vi "Apply Module Limits Fixed.vi"(8 "error in":errorcluster, 11 "3300 in":refnum<class "3300.lvclass">) -> (0 "error out":errorcluster, 3 "3300 out":refnum<class "3300.lvclass">)   [LabVIEW 2019, in "3300.lvlib" / "3300.lvclass"]
uses:
  Library/3300.lvclass
  C:/Users/Public/Documents/Development/builds/Instruments/Electronic Load.lvlibp/Library/Electronic Load.lvclass
  builds/Instruments/Electronic Load.lvlibp/Private/GUI/Read Settings_Ref.vi
  Module Support/Access Module Limits.vi
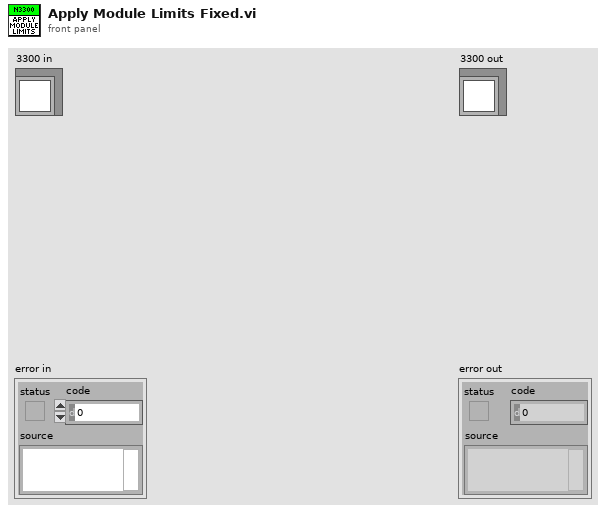
[diagram p1: front panel]
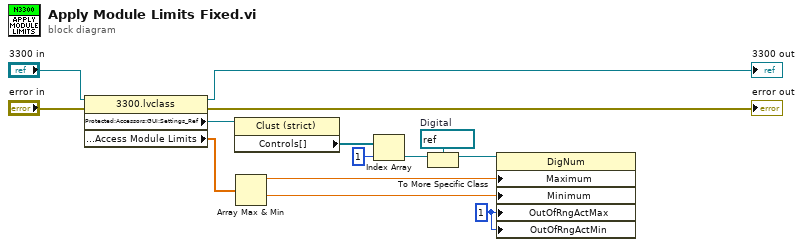
[diagram p0: block diagram]
diagram:
  w1 = u8 1 ("Response to Value Outside Limits:Maximum")
  w6 = refnum<vi> refnum  # Digital
  n1 = property class="3300.lvclass"(reference="3300 in", error in="error in") -> (reference out=→"3300 out":refnum<class "3300.lvclass">, error out=→"error out":errorcluster, "Protected:Accessors:GUI:Settings_Ref"=w11:refnum<vi>, "Private:Accessors:Access Module Limits"=w12:dbl[])
  n2 = property class="Clust (strict)"(reference=w11) -> ("Controls[]"=w10:refnum<vi>[])  [unwired: 1 in, 2 out]
  n3 = Array Max & Min(array=w12) -> (max value=w5:dbl, min value=w4:dbl)  [unwired: 2 out]
  n4 = Index Array(array=w10, index=1) -> (element=w8:refnum<vi>)
  n5 = To More Specific Class(target class=w6, reference=w8) -> (specific class reference=w7:refnum<vi>)  [unwired: 1 in, 1 out]
  n6 = property class="DigNum"(reference=w7, "Maximum"=w5, "Minimum"=w4, "OutOfRngActMax"=w1, "OutOfRngActMin"=w1) -> ()  [unwired: 1 in, 2 out]
